vi "Generate New File.vi"(8 "error in":errorcluster, 11 "File Obs in":refnum<class "File Observer.lvclass">) -> (0 "error out":errorcluster, 2 "File Ref Out":refnum<file>, 3 "File Obs out":refnum<class "File Observer.lvclass">)   [LabVIEW 2015, in "File Observer.lvclass"]
doc: "Generate a New File for use by the observer based on the caller defined File Name and Data Path. If there is a file open, close it."
uses:
  File Observer.lvclass
  File Observer.lvclass/File Observer.ctl
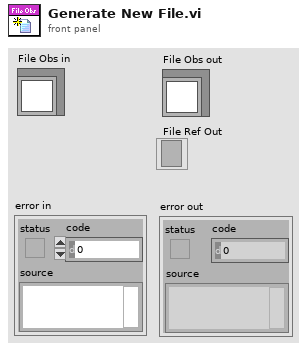
[diagram p1: front panel]
types:
  T1 = enum16{"open", "replace", "create", "open or create", "replace or create", "replace or create with confirmation"}
  T2 = typedef "LVDateTimeRec.ctl" = cluster{"fractional second":dbl, "second":i32, "minute":i32, "hour":i32, "day of month":i32, "month":i32, "year":i32, "day of week":i32, "day of year":i32, "DST":i32}
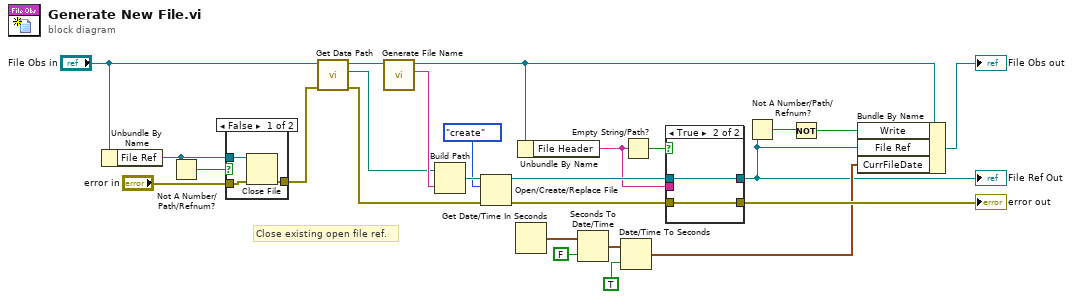
[diagram p0: block diagram]
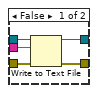
[diagram p2: hidden frame]
diagram:
  # "Close existing open file ref."
  n1 = Unbundle By Name("File Obs in") -> ("File Ref"=w17:refnum<file>)
  n2 = Not A Number/Path/Refnum?(number/path/refnum=w17) -> (NaN/Path/Refnum?=w18:bool)
  n3 = case shown="False" w18 {
    tunnel: w17 -> [w29 _]
    tunnel: "error in" -> [w28 w30]
    tunnel: [w27 w30] -> w15
    frame False {
      n4 = Close File(refnum=w29, error in=w28) -> (error out=w27:errorcluster)  [unwired: 1 out]
    }
    frame True {
    }
  }
  n5 = call-dynamic "Get Data Path.vi"("error in"=w15, "File Observer in"="File Obs in") -> ("error out"=w23:errorcluster, "path out"=w20:path, "File Observer out"=w21:refnum<class "File Observer.lvclass">)  [unwired: 7 in]
  n6 = call-dynamic "Generate File Name.vi"("File Obs in"=w21) -> ("File Name"=w22:string, "File Obs out"=w14:refnum<class "File Observer.lvclass">)  [unwired: 9 in]
  n7 = Build Path(base path=w20, name or relative path=w22) -> (appended path=w25:path)
  n8 = Open/Create/Replace File(file path (use dialog)=w25, error in=w23, operation (0:open)=T1."create") -> (refnum out=w13:refnum<file>, error out=w12:errorcluster)  [unwired: 4 out]
  n9 = Get Date/Time In Seconds() -> (seconds since 1Jan1904=w8:timestamp)
  n10 = Unbundle By Name(w14) -> ("File Header"=w9:string)
  n11 = Seconds To Date/Time(time stamp (now)=w8, to UTC (F)=FALSE) -> (date time rec=w5:T2)
  n12 = Date/Time To Seconds(1:TRUE ("is UTC (F)"), 2:w5) -> (0:w4:timestamp)
  n13 = Empty String/Path?(string/path=w9) -> (empty?=w10:bool)
  n14 = case shown="True" w10 {
    tunnel: w13 -> [w35 w37]
    tunnel: w12 -> [w34 w36]
    tunnel: [w33 w37] -> w3
    tunnel: [w32 w36] -> w11
    tunnel: w9 -> [w31 _]
    frame False {
      n15 = Write to Text File(file (use dialog)=w35, text=w31, error in=w34) -> (refnum out=w33:refnum<file>, error out=w32:errorcluster)  [unwired: 1 in, 1 out]
    }
    frame True {
    }
  }
  "error out" <- w11
  "File Ref Out" <- w3
  n16 = Not A Number/Path/Refnum?(number/path/refnum=w3) -> (NaN/Path/Refnum?=w2:bool)
  n17 = Not(x=w2) -> (.not. x?=w1:bool)
  n18 = Bundle By Name(cluster=w14, "Write"=w1, "File Ref"=w3, "CurrFileDate"=w4) -> (→"File Obs out":refnum<class "File Observer.lvclass">)
